vi "gz (SubVI).vi"(6 "Array in":dbl[](array[numeric]), 9 "Array 3":dbl[](array[numeric]), 10 "Array 4":dbl[](array[numeric]), 11 "Array 5":dbl[](array[numeric])) -> (3 "Array out":dbl[](array[numeric]))   [LabVIEW 2011]
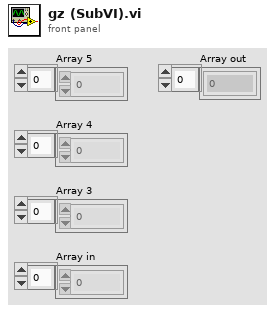
[diagram p1: front panel]
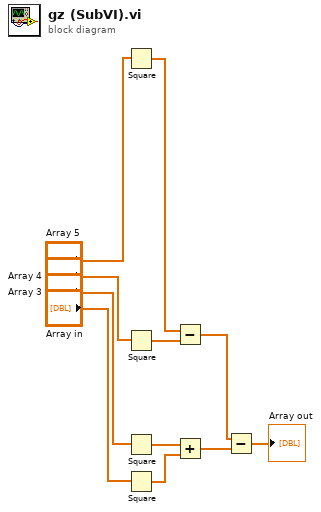
[diagram p0: block diagram]
diagram:
  n1 = Square(x="Array 5") -> (x^2=w5:dbl[])
  n2 = Square(x="Array 4") -> (x^2=w6:dbl[])
  n3 = Square(x="Array 3") -> (x^2=w7:dbl[])
  n4 = Square(x="Array in") -> (x^2=w8:dbl[])
  n5 = Subtract(x=w5, y=w6) -> (x-y=w9:dbl[])
  n6 = Add(x=w7, y=w8) -> (x+y=w10:dbl[])
  n7 = Subtract(x=w9, y=w10) -> (x-y=→"Array out":dbl[])
